vi "UACreateServer.vi"(8 "error in (no error)":errorcluster, 11 "Server config info":T1) -> (0 "error out":errorcluster, 1 "server endpoint URL":string, 2 "OPC UA server refnum out":refnum<k21>, 3 "Server config info (dup)":T1)   [LabVIEW 2014, in "OPCUA XML.lvlib"]
uses:
  OPCUA XML.lvlib
  DEF-Server Config Data.ctl
  <vilib>/OPCUA/NI OPC UA Server.lvlib
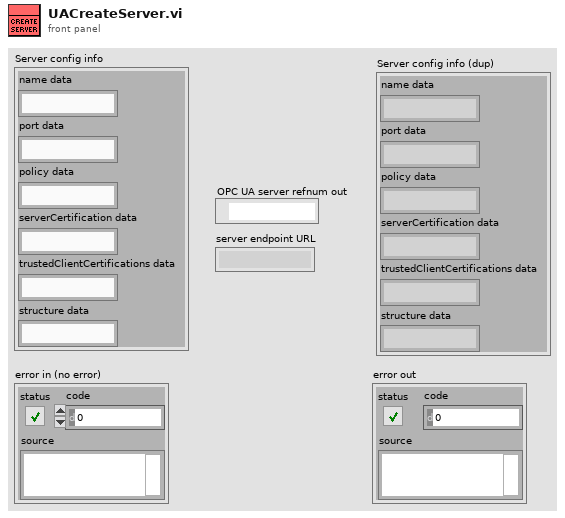
[diagram p1: front panel]
types:
  T1 = typedef "OPCUA XML.lvlib/DEF-Server Config Data.ctl" = cluster{"name data":string, "port data":string, "policy data":string, "serverCertification data":string, "trustedClientCertifications data":string, "structure data":string}
  T2 = typedef "supported security policies.ctl" = cluster{"None":bool, "Sign with Basic128Rsa125":bool, "Sign and Encrypt with Basic128Rsa125":bool, "Sign with Basic256":bool, "Sign and Encrypt with Basic256":bool}
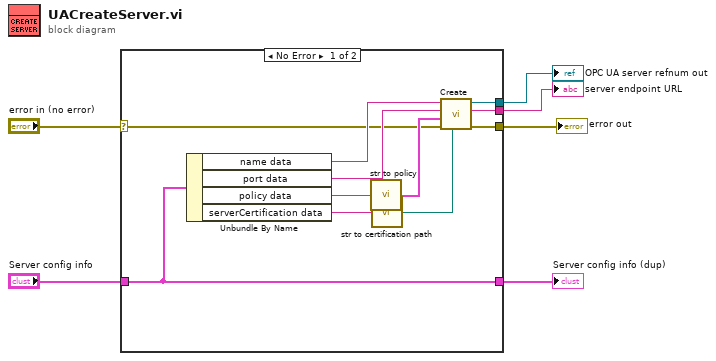
[diagram p0: block diagram]
diagram:
  n1 = case shown="No Error" "error in (no error)" {
    selector: "error in (no error)" -> [w8 w19]
    tunnel: [w17 w19] -> w6
    tunnel: [w10 _] -> w5
    tunnel: [w9 _] -> w4
    tunnel: "Server config info" -> [w7 w18]
    tunnel: [w7 w18] -> w1
    frame No Error {
      n2 = Unbundle By Name(w7) -> ("name data"=w13:string, "port data"=w14:string, "policy data"=w15:string, "serverCertification data"=w16:string)
      n3 = call "str to policy.vi"("String"=w15) -> ("supported security policies (None)"=w11:T2)  [unwired: 6 in]
      n4 = call "str to certification path.vi"("node text"=w16) -> ("File Path Control"=w12:path)  [unwired: 4 in]
      n5 = call <vilib>:"Create.vi"("server certificate file"=w12, "error in (no error)"=w8, "supported security policies (None)"=w11, "TCP port (49580)"=w14, "OPC UA server name"=w13) -> ("error out"=w17:errorcluster, "server endpoint URL"=w9:string, "OPC UA server refnum out"=w10:refnum<k21>)  [unwired: 4 in]
    }
    frame Error {
    }
  }
  "error out" <- w6
  "OPC UA server refnum out" <- w5
  "server endpoint URL" <- w4
  "Server config info (dup)" <- w1
